vi "constructor.vi"(8 "error in (no error)":errorcluster, 10 "camera settings":string) -> (0 "error out":errorcluster, 3 "CamaraSettings out":refnum<class "CamaraSettings.lvclass">)   [LabVIEW 2009, in "Tools.lvlib" / "Settings.lvlib" / "CamaraSettings.lvclass"]
uses:
  CamaraSettings.lvclass
  PixelFlySettings/PixelflySettings.lvclass
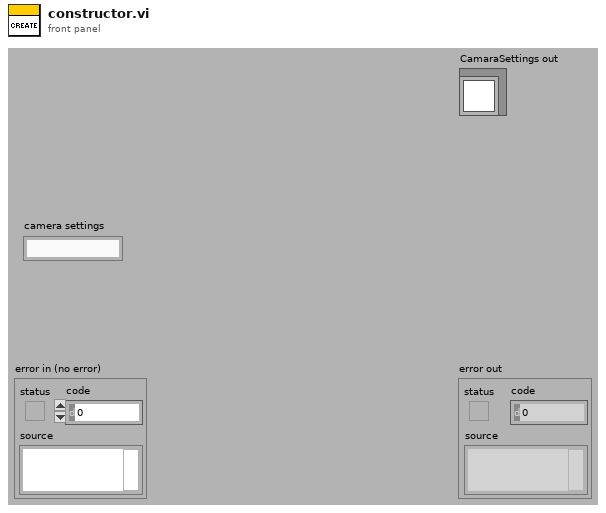
[diagram p1: front panel]
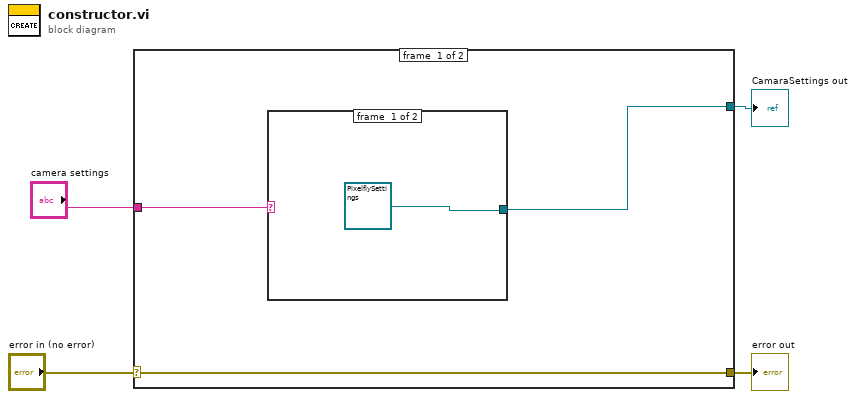
[diagram p0: block diagram]
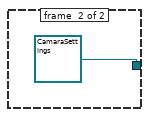
[diagram p2: hidden frame]
diagram:
  n1 = case shown="No Error" "error in (no error)" {
    selector: "error in (no error)" -> [w7 w10]
    tunnel: [w7 w10] -> w3
    tunnel: "camera settings" -> [w6 _]
    tunnel: [w5 _] -> w1
    frame #0 {
      n2 = case shown="Default" w6 {
        tunnel: [refnum<class "PixelflySettings.lvclass"> refnum ("Tools.lvlib:Settings.lvlib:PixelflySettings.lvclass") refnum<class "CamaraSettings.lvclass"> refnum ("Tools.lvlib:Settings.lvlib:CamaraSettings.lvclass")] -> w5
        frame #0 {
        }
        frame #1 {
        }
      }
    }
    frame #1 {
    }
  }
  "error out" <- w3
  "CamaraSettings out" <- w1
